vi "TESTC.vi"(8 "error in":errorcluster, 10 "Image In":T1, 11 "Session In":T2="cam1") -> (0 "x != 0?":bool, 1 "Image Out":T1(plugin-control), 2 "dcolor":i32, 3 "ucolor":i32, 4 "Classes (Color Classification 2)":string[](array[string]), 5 "Classes (Color Classification 1)":string[](array[string]), 6 "error out":errorcluster)   [LabVIEW 2018]
uses:
  <vilib>/userdefined/High Color/IMAQdx.ctl
  <vilib>/vision/Image Controls.llb/IMAQ Image.ctl
  <vilib>/vision/driver/NI_Vision_Acquisition_Software.lvlib
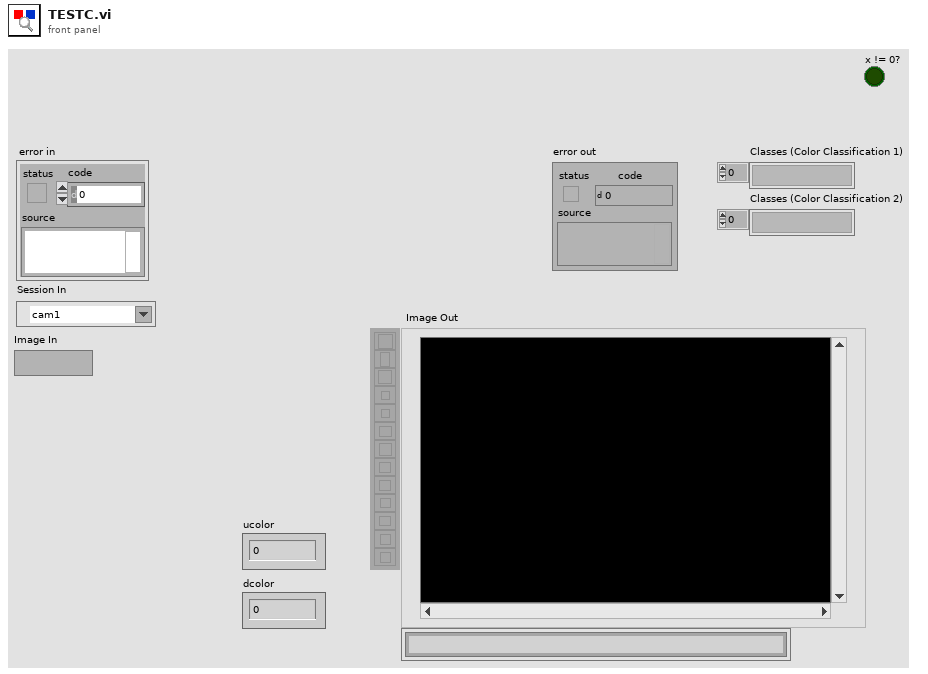
[diagram p1: front panel]
types:
  T1 = typedef "IMAQ Image.ctl" = refnum<image>
  T2 = typedef "IMAQdx.ctl" = refnum<k21>
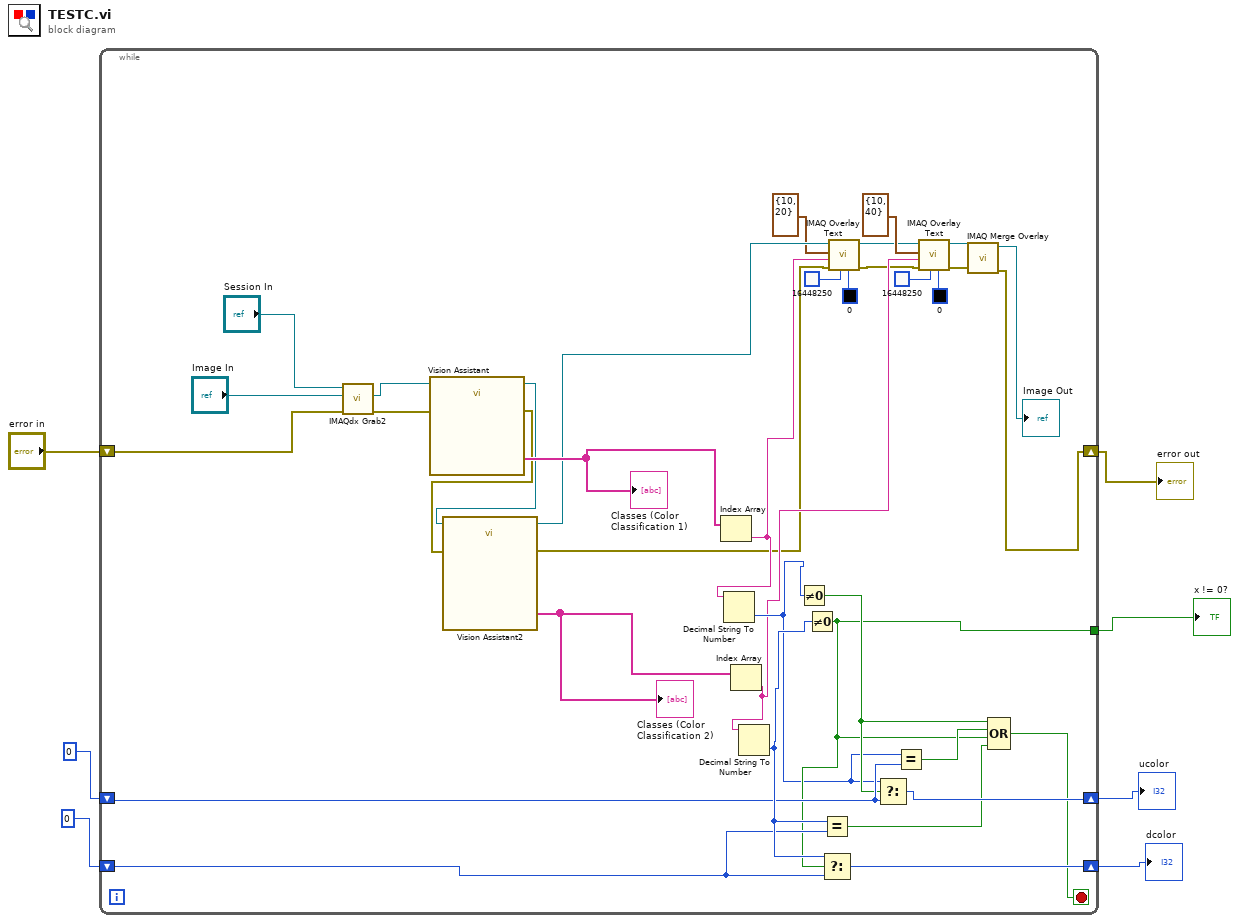
[diagram p0: block diagram]
diagram:
  n1 = while {
    tunnel: [w33] -> w7
    shift-right: [w37] -> w4
    shift-left: 0 -> [w38]
    shift-right: [w41] -> w3
    shift-left: 0 -> [w39]
    shift-right: [w10] -> w1
    shift-left: "error in" -> [w14]
    stop <- w32 stop-if-true
    n2 = call <vilib>:"IMAQdx Grab2.vi"("error in"=w14, "Image In"="Image In", "Session In"="Session In") -> ("error out"=w31:errorcluster, "Image Out"=w28:T1)  [unwired: 5 in, 2 out]
    n3 = call "Vision Assistant"("Image In"=w28, "error in"=w31) -> ("Image Out"=w27:T1, "Classes (Color Classification 1)"=w43:string[], "error out"=w15:errorcluster)  [unwired: 22 in, 1 out]
    "Classes (Color Classification 1)" <- w43
    n4 = call "Vision Assistant2"("Image In"=w27, "error in"=w15) -> ("Image Out"=w25:T1, "Classes (Color Classification 2)"=w42:string[], "error out"=w9:errorcluster)  [unwired: 22 in, 1 out]
    "Classes (Color Classification 2)" <- w42
    n5 = Index Array(array=w43) -> (element=w24:string)  [unwired: 1 in]
    n6 = Decimal String To Number(string=w24) -> (number=w26:i32)  [unwired: 2 in, 1 out]
    n7 = Index Array(array=w42) -> (element=w16:string)  [unwired: 1 in]
    n8 = Decimal String To Number(string=w16) -> (number=w40:i32)  [unwired: 2 in, 1 out]
    n9 = Not Equal To 0?(x=w26) -> (x != 0?=w34:bool)
    n10 = Not Equal To 0?(x=w40) -> (x != 0?=w33:bool)
    n11 = Equal?(x=w40, y=w39) -> (x = y?=w35:bool)
    n12 = Select(t=w40, s=w33, f=w39) -> (s? t:f=w41:i32)
    n13 = call "IMAQ Overlay Text"("BG Color (Transparent)"=u32 0, "Text Color (black)"=u32 16448250, "error in (no error)"=w9, "String"=w24, "Origin"=cluster{"X":i32, "Y":i32} {"X"=10, "Y"=20}, "Image"=w25) -> ("error out"=w11:errorcluster, "Image Out"=w17:T1)  [unwired: 4 in]
    n14 = Select(t=w26, s=w34, f=w38) -> (s? t:f=w37:i32)
    n15 = Equal?(x=w26, y=w38) -> (x = y?=w36:bool)
    n16 = call "IMAQ Overlay Text"("BG Color (Transparent)"=u32 0, "Text Color (black)"=u32 16448250, "error in (no error)"=w11, "String"=w16, "Origin"=cluster{"X":i32, "Y":i32} {"X"=10, "Y"=40}, "Image"=w17) -> ("error out"=w13:errorcluster, "Image Out"=w12:T1)  [unwired: 4 in]
    n17 = call "IMAQ Merge Overlay"("error in (no error)"=w13, "Image Src"=w12) -> ("error out"=w10:errorcluster, "Image Dst Out"=→"Image Out":T1)  [unwired: 8 in]
    n18 = Compound Arithmetic op=OR(w34, w36, w33, w35) -> (w32:bool)
  }
  "x != 0?" <- w7
  "ucolor" <- w4
  "dcolor" <- w3
  "error out" <- w1
